vi "Robot Turning.vi"() -> ()   [LabVIEW 2012]
panel:
  in  "Robot Turning?":bool
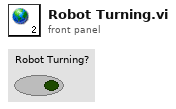
[diagram p1: front panel]
diagram:
